vi "Wait For (str) (SubVI).vi"(9 "字符串":string, 10 "queue out":refnum<queue>, 11 ".NET引用句柄输入":refnum<k24>) -> (0 "错误输出":errorcluster)   [LabVIEW 2019, in "Take Seq.lvlib"]
uses:
  Take Seq.lvlib
  config.ctl
  Instrument.ctl
  lib/QDInstrument.dll
  SubVI.lvlib
panel:
  # "(真是通道1，假是通道2)"
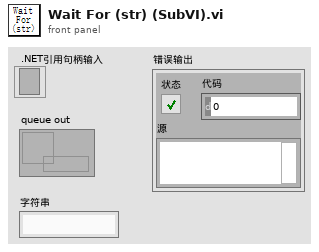
[diagram p1: front panel]
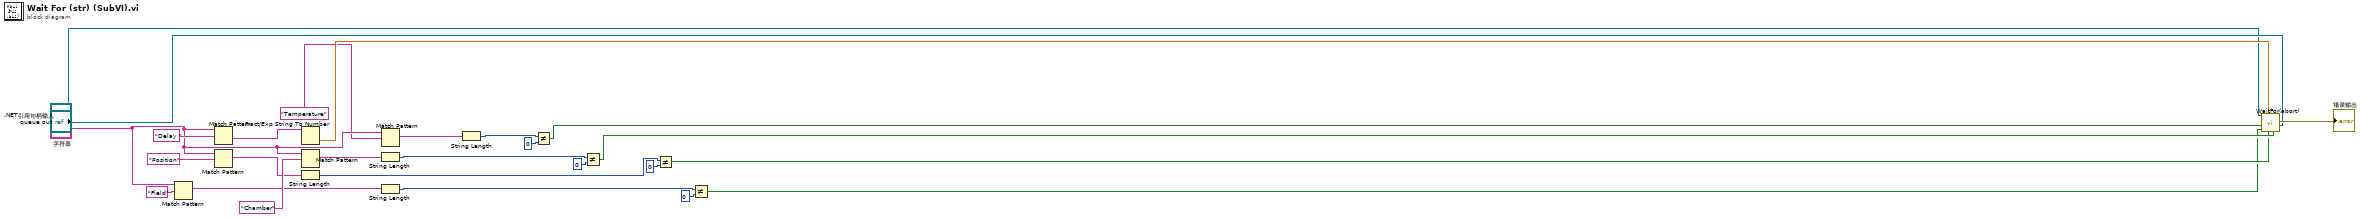
[diagram p0: block diagram]
diagram:
  n1 = Match Pattern(string="字符串", regular expression="Field" ("正则表达式")) -> (match substring=w6:string)  [unwired: 1 in, 3 out]
  n2 = Match Pattern(string="字符串", regular expression="Delay " ("正则表达式")) -> (after substring=w22:string)  [unwired: 1 in, 3 out]
  n3 = Match Pattern(string="字符串", regular expression="Position" ("正则表达式")) -> (match substring=w9:string)  [unwired: 1 in, 3 out]
  n4 = Fract/Exp String To Number(string=w22) -> (number=w23:dbl)  [unwired: 3 in, 1 out]
  n5 = Match Pattern(string="字符串", regular expression="Chamber" ("正则表达式")) -> (match substring=w12:string)  [unwired: 1 in, 3 out]
  n6 = String Length(string=w9) -> (length=w10:i32)
  n7 = Match Pattern(string="字符串", regular expression="Temperature" ("正则表达式")) -> (match substring=w2:string)  [unwired: 1 in, 3 out]
  n8 = String Length(string=w12) -> (length=w13:i32)
  n9 = String Length(string=w6) -> (length=w7:i32)
  n10 = String Length(string=w2) -> (length=w3:i32)
  n11 = Not Equal?(x=w3, y=0) -> (x != y?=w5:bool)
  n12 = Not Equal?(x=w13, y=0) -> (x != y?=w25:bool)
  n13 = Not Equal?(x=w10, y=0) -> (x != y?=w24:bool)
  n14 = Not Equal?(x=w7, y=0) -> (x != y?=w19:bool)
  n15 = call "WaitFor(abort).vi"("config"="queue out", "Wait For Chamber"=w25, "Wait For Position"=w24, "Delay"=w23, "Wait For Field"=w19, "Wait For Temperature"=w5, "Instrument Ref In"=".NET引用句柄输入") -> ("error out"=→"错误输出":errorcluster)  [unwired: 3 in, 1 out]
